vi "Control loop cluster to String.vi"(11 "Control Loop":T1) -> (3 "Data to send":string="EXCT:TYPE:Unipolar:MAG:10.00:EXCT:NICK:MB1.T1:LOOP:AUX:None:PSET:1.0:HTR:None:ISET:1.0:HAUT:Manual:HSET:0.0:PIDT:Manual:DSET:1.0:TSET:0K:LVL:MB1.T1:LOOP:MAN:HVER:0:FVER:20.6:SERL:102750119:MAN:CAL:OFFS:0.0000:COLD:1.0000:INT:Linear:SCAL:1.0000:FILE:RP5.DAT:HOTL:1023.1500:CAL:TYPE:PTC:SIG:VOLT:1405.9mV:CURR:10µA:TEMP:1023.15K:POWR:14.059µW:RES:140590?:SLOP:137.409?/K:FLOW:NOT_FOUND:SIG:TEMP\n")   [LabVIEW 2015, in "Mercury iXX.lvlib" / "Control Loop.lvlib"]
uses:
  Control Loop.lvlib
  Temperature/Controls/Loop Cluster.ctl
  Temperature.lvlib
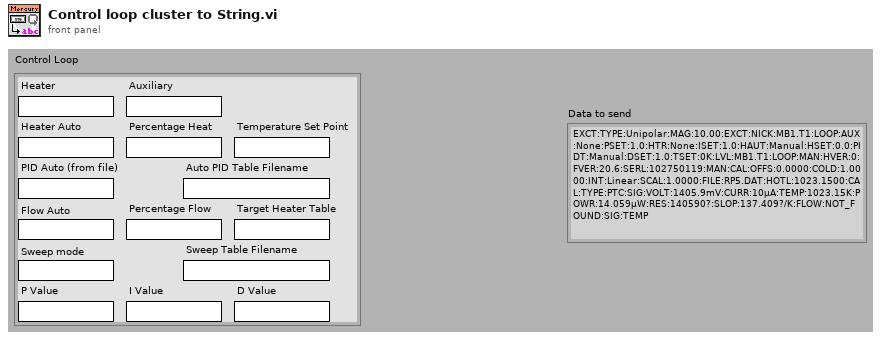
[diagram p1: front panel]
types:
  T1 = typedef "Mercury iXX.lvlib/Temperature.lvlib/Loop Cluster.ctl" = cluster{"Heater":string, "Auxiliary":string, "Heater Auto":string, "Percentage Heat":string, "Temperature Set Point":string, "PID Auto (from file)":string, "P Value":string, "I Value":string, "D Value":string, "Auto PID Table Filename":string, "Flow Auto":string, "Target Heater Table":string, "Sweep mode":string, "Sweep Table Filename":string, "Percentage Flow":string}
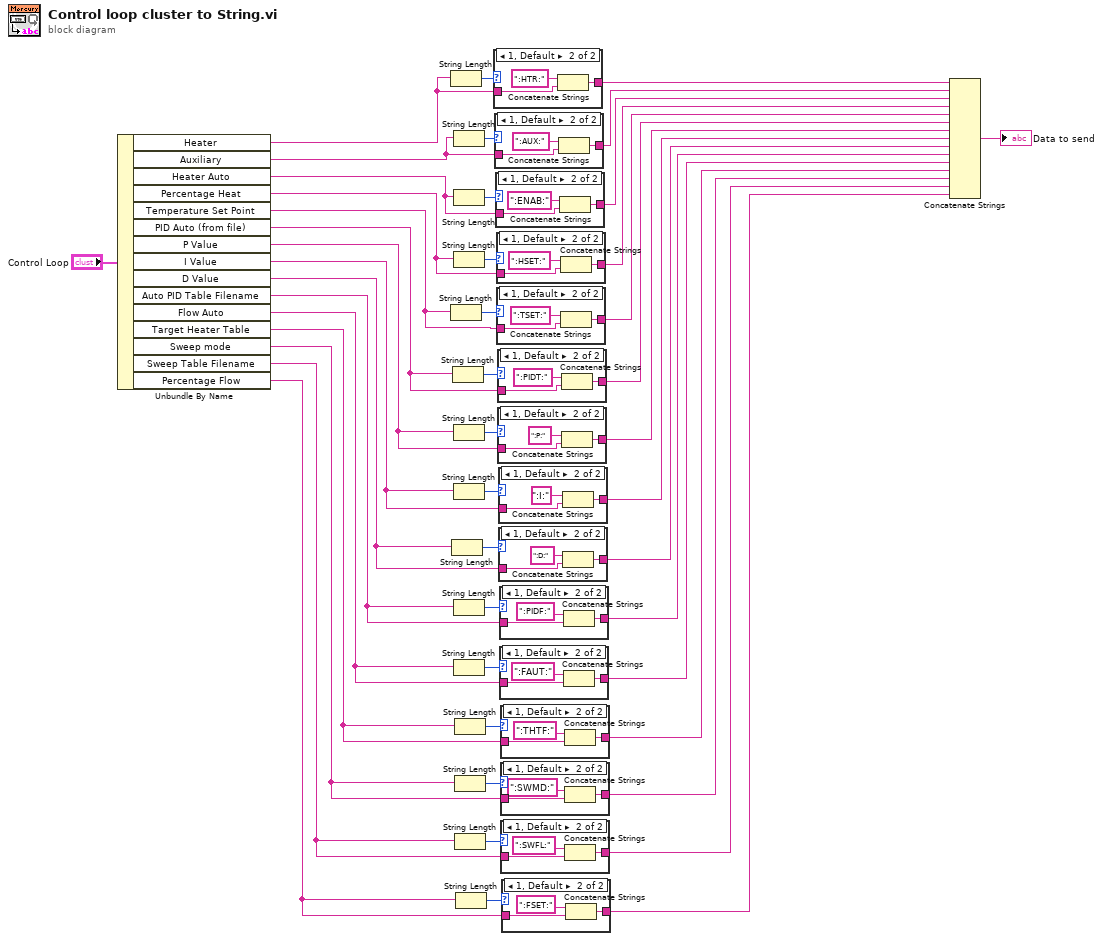
[diagram p0: block diagram]
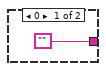
[diagram p2: hidden frame]
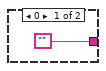
[diagram p3: hidden frame]
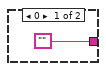
[diagram p4: hidden frame]
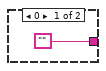
[diagram p5: hidden frame]
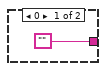
[diagram p6: hidden frame]
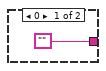
[diagram p7: hidden frame]
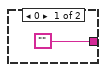
[diagram p8: hidden frame]
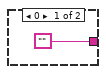
[diagram p9: hidden frame]
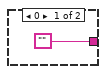
[diagram p10: hidden frame]
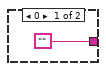
[diagram p11: hidden frame]
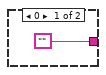
[diagram p12: hidden frame]
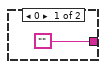
[diagram p13: hidden frame]
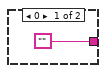
[diagram p14: hidden frame]
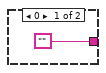
[diagram p15: hidden frame]
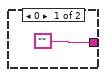
[diagram p16: hidden frame]
diagram:
  n1 = Unbundle By Name("Control Loop") -> ("Heater"=w45:string, "Auxiliary"=w43:string, "Heater Auto"=w32:string, "Percentage Heat"=w31:string, "Temperature Set Point"=w30:string, "PID Auto (from file)"=w29:string, "P Value"=w28:string, "I Value"=w27:string, "D Value"=w26:string, "Auto PID Table Filename"=w25:string, "Flow Auto"=w13:string, "Target Heater Table"=w12:string, "Sweep mode"=w8:string, "Sweep Table Filename"=w7:string, "Percentage Flow"=w2:string)
  n2 = String Length(string=w45) -> (length=w46:i32)
  n3 = String Length(string=w30) -> (length=w37:i32)
  n4 = String Length(string=w26) -> (length=w33:i32)
  n5 = String Length(string=w29) -> (length=w36:i32)
  n6 = String Length(string=w43) -> (length=w44:i32)
  n7 = String Length(string=w32) -> (length=w38:i32)
  n8 = String Length(string=w31) -> (length=w39:i32)
  n9 = String Length(string=w28) -> (length=w34:i32)
  n10 = String Length(string=w27) -> (length=w35:i32)
  n11 = String Length(string=w25) -> (length=w16:i32)
  n12 = String Length(string=w13) -> (length=w14:i32)
  n13 = String Length(string=w12) -> (length=w15:i32)
  n14 = String Length(string=w8) -> (length=w9:i32)
  n15 = String Length(string=w7) -> (length=w3:i32)
  n16 = String Length(string=w2) -> (length=w4:i32)
  n17 = case shown="1, Default" w46 {
    tunnel: w45 -> [_ w50]
    tunnel: ["" w51] -> w42
    frame 0 {
    }
    frame 1, Default {
      n18 = Concatenate Strings(":HTR:" ("string"), w50) -> (w51:string)
    }
  }
  n19 = case shown="1, Default" w44 {
    tunnel: w43 -> [_ w54]
    tunnel: ["" w55] -> w41
    frame 0 {
    }
    frame 1, Default {
      n20 = Concatenate Strings(":AUX:" ("string"), w54) -> (w55:string)
    }
  }
  n21 = case shown="1, Default" w38 {
    tunnel: w32 -> [_ w58]
    tunnel: ["" w59] -> w24
    frame 0 {
    }
    frame 1, Default {
      n22 = Concatenate Strings(":ENAB:" ("string"), w58) -> (w59:string)
    }
  }
  n23 = case shown="1, Default" w39 {
    tunnel: w31 -> [_ w62]
    tunnel: ["" w63] -> w23
    frame 0 {
    }
    frame 1, Default {
      n24 = Concatenate Strings(":HSET:" ("string"), w62) -> (w63:string)
    }
  }
  n25 = case shown="1, Default" w37 {
    tunnel: w30 -> [_ w66]
    tunnel: ["" w67] -> w22
    frame 0 {
    }
    frame 1, Default {
      n26 = Concatenate Strings(":TSET:" ("string"), w66) -> (w67:string)
    }
  }
  n27 = case shown="1, Default" w36 {
    tunnel: w29 -> [_ w70]
    tunnel: ["" w71] -> w21
    frame 0 {
    }
    frame 1, Default {
      n28 = Concatenate Strings(":PIDT:" ("string"), w70) -> (w71:string)
    }
  }
  n29 = case shown="1, Default" w34 {
    tunnel: w28 -> [_ w74]
    tunnel: ["" w75] -> w20
    frame 0 {
    }
    frame 1, Default {
      n30 = Concatenate Strings(":P:" ("string"), w74) -> (w75:string)
    }
  }
  n31 = case shown="1, Default" w35 {
    tunnel: w27 -> [_ w78]
    tunnel: ["" w79] -> w19
    frame 0 {
    }
    frame 1, Default {
      n32 = Concatenate Strings(":I:" ("string"), w78) -> (w79:string)
    }
  }
  n33 = case shown="1, Default" w33 {
    tunnel: w26 -> [_ w82]
    tunnel: ["" w83] -> w18
    frame 0 {
    }
    frame 1, Default {
      n34 = Concatenate Strings(":D:" ("string"), w82) -> (w83:string)
    }
  }
  n35 = case shown="1, Default" w16 {
    tunnel: w25 -> [_ w86]
    tunnel: ["" w87] -> w17
    frame 0 {
    }
    frame 1, Default {
      n36 = Concatenate Strings(":PIDF:" ("string"), w86) -> (w87:string)
    }
  }
  n37 = case shown="1, Default" w14 {
    tunnel: w13 -> [_ w90]
    tunnel: ["" w91] -> w11
    frame 0 {
    }
    frame 1, Default {
      n38 = Concatenate Strings(":FAUT:" ("string"), w90) -> (w91:string)
    }
  }
  n39 = case shown="1, Default" w15 {
    tunnel: w12 -> [_ w94]
    tunnel: ["" w95] -> w10
    frame 0 {
    }
    frame 1, Default {
      n40 = Concatenate Strings(":THTF:" ("string"), w94) -> (w95:string)
    }
  }
  n41 = case shown="1, Default" w9 {
    tunnel: w8 -> [_ w98]
    tunnel: ["" w99] -> w6
    frame 0 {
    }
    frame 1, Default {
      n42 = Concatenate Strings(":SWMD:" ("string"), w98) -> (w99:string)
    }
  }
  n43 = case shown="1, Default" w3 {
    tunnel: w7 -> [_ w102]
    tunnel: ["" w103] -> w5
    frame 0 {
    }
    frame 1, Default {
      n44 = Concatenate Strings(":SWFL:" ("string"), w102) -> (w103:string)
    }
  }
  n45 = case shown="1, Default" w4 {
    tunnel: w2 -> [_ w106]
    tunnel: ["" w107] -> w1
    frame 0 {
    }
    frame 1, Default {
      n46 = Concatenate Strings(":FSET:" ("string"), w106) -> (w107:string)
    }
  }
  n47 = Concatenate Strings(w42, w41, w24, w23, w22, w21, w20, w19, w18, w17, w11, w10, w6, w5, w1) -> (→"Data to send":string)
